vi "Send_Data_DAQ.vi"(8 "error in":errorcluster, 9 "AI Trig":bool, 10 "AI duration (ms)":i32=100, 11 "Digital Ports":tag="Dev1/port0") -> (0 "error out":errorcluster, 2 "data":waveform(dbl))   [LabVIEW 2021]
uses:
  <vilib>/DAQmx/write.llb/DAQmx Write (Digital 1D U32 1Chan NSamp).vi
  <vilib>/DAQmx/read.llb/DAQmx Read (Analog Wfm 1Chan NSamp).vi
  <vilib>/DAQmx/create/channels.llb/DAQmx Create Channel (DO-Digital Output).vi
  <vilib>/DAQmx/create/channels.llb/DAQmx Create Channel (CO-Pulse Generation-Ticks).vi
  <vilib>/DAQmx/configure/timing.llb/DAQmx Timing (Implicit).vi
  <vilib>/DAQmx/create/channels.llb/DAQmx Create Channel (AI-Voltage-Basic).vi
  <vilib>/DAQmx/configure/timing.llb/DAQmx Timing (Sample Clock).vi
  <vilib>/DAQmx/configure/trigger.llb/DAQmx Start Trigger (None).vi
  <vilib>/DAQmx/configure/trigger.llb/DAQmx Start Trigger (Analog Edge).vi
  Global_DAQ.vi
  <vilib>/DAQmx/create/channels.llb/DAQmx Create Channel (CO-Pulse Generation-Frequency).vi
  <vilib>/DAQmx/miscellaneous.llb/DAQmx Fill In Error Info.vi
  <vilib>/Utility/error.llb/Error Cluster From Error Code.vi
  <vilib>/ErrorRing/Error Ring.xnode
panel:
  out "Waveform Graph":waveform(dbl)(graph)
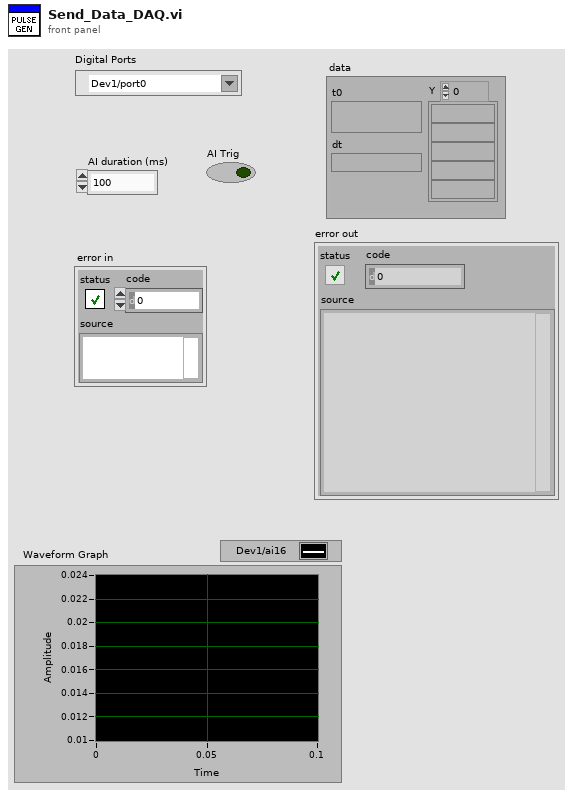
[diagram p1: front panel]
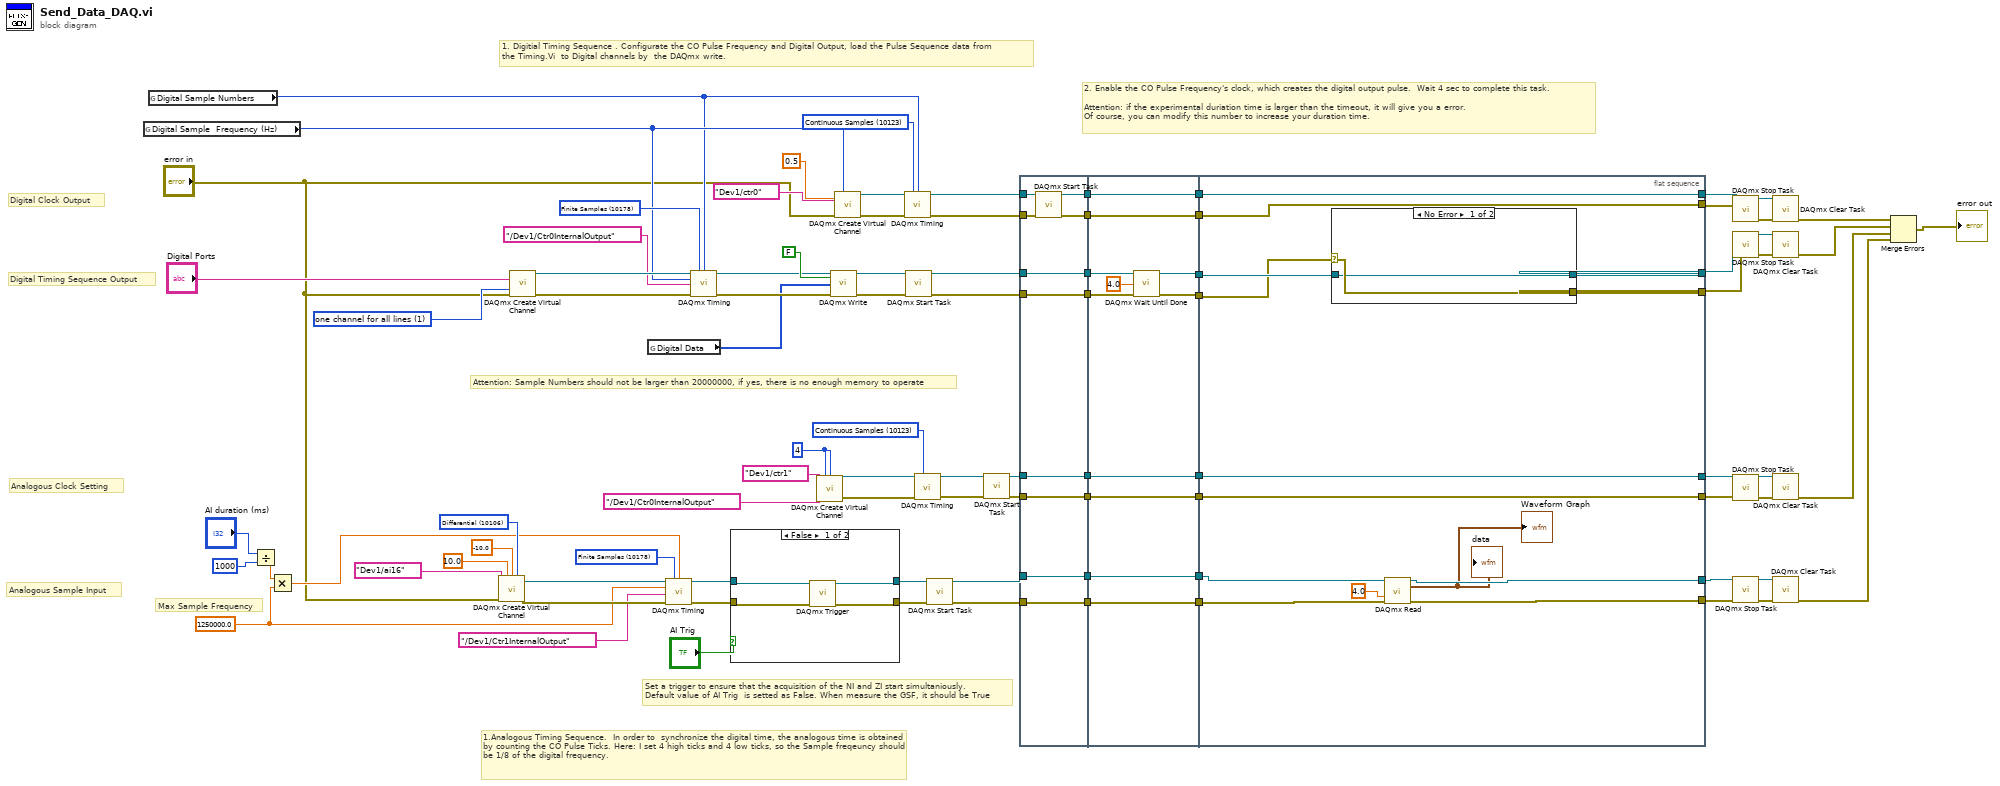
[diagram p0: block diagram]
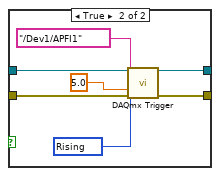
[diagram p2: hidden frame]
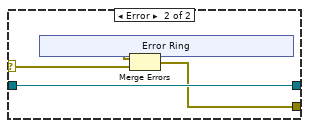
[diagram p3: hidden frame]
diagram:
  w35 = 1250000.0 ("rate")
  w38 = 10106 items=["Default"=-1, "RSE"=10083, "NRSE"=10078, "Differential"=10106, "Pseudodifferential"=12529] ("input terminal configuration")
  w39 = 10178 items=["Finite Samples"=10178, "Continuous Samples"=10123, "Hardware Timed Single Point"=12522] ("sample mode")
  w52 = 10123 items=["Finite Samples"=10178, "Continuous Samples"=10123, "Hardware Timed Single Point"=12522] ("sample mode")
  w53 = u32 4 ("low ticks")
  w81 = 10178 items=["Finite Samples"=10178, "Continuous Samples"=10123, "Hardware Timed Single Point"=12522] ("sample mode")
  w82 = 1 items=["one channel for each line", "one channel for all lines"] ("line grouping")
  w87 = 10123 items=["Finite Samples"=10178, "Continuous Samples"=10123, "Hardware Timed Single Point"=12522] ("sample mode")
  # "Analogous Sample Input"
  # "Analogous Clock Setting"
  # "Digital Timing Sequence Output"
  # "Digital Clock Output"
  # "Set a trigger to ensure that the acquisition of the NI and ZI start simultaniously.\nDefault value of AI Trig  is setted as False. When measure the GSF, it should be True"
  # "1.Analogous Timing Sequence.  In order to  synchronize the digital time, the analogous time is obtained by counting the CO Pulse Ticks. Here: I set 4 high ticks and 4 low ticks, so the Sample freqeuncy should be 1/8 of the digital frequency."
  # "Max Sample Frequency"
  # "Attention: Sample Numbers should not be larger than 20000000, if yes, there is no enough memory to operate"
  # "2. Enable the CO Pulse Frequency's clock, which creates the digital output pulse.  Wait 4 sec to complete this task.    \n\nAttention: if the experimental duriation time is larger than the timeout, it will give you a error.\nOf course, you can modify this number to increase your duration time."
  # "1. Digitial Timing Sequence . Configurate the CO Pulse Frequency and Digital Output, load the Pulse Sequence data from\nthe Timing.Vi  to Digital channels by  the DAQmx write."
  n1 = global read "Global_DAQ.vi" "Digital Sample  Frequency (Hz)"() -> (w64:u32)
  n2 = global read "Global_DAQ.vi" "Digital Sample Numbers"() -> (w61:u32)
  n3 = Divide(x="AI duration (ms)", y=1000) -> (x/y=w36:dbl)
  n4 = Multiply(x=w36, y=w35) -> (x*y=w33:dbl)
  n5 = call-poly <vilib>:"DAQmx Create Virtual Channel.vi"("maximum value"=10.0, "minimum value"=-10.0, "input terminal configuration"=w38, "physical channels"=tag "Dev1/ai16", "error in"="error in") -> ("task out"=w46:refnum<k21>, "error out"=w45:errorcluster)  [unwired: 9 in]
  n6 = call-poly <vilib>:"DAQmx Create Virtual Channel.vi"("lines"="Digital Ports", "line grouping"=w82, "error in"="error in") -> ("task out"=w86:refnum<k21>, "error out"=w85:errorcluster)  [unwired: 11 in]
  n7 = global read "Global_DAQ.vi" "Digital Data"() -> (w58:u32[])
  n8 = call-poly <vilib>:"DAQmx Timing.vi"("task/channels in"=w46, "sample mode"=w39, "samples per channel"=w33, "rate"=w35, "source"=tag "/Dev1/Ctr1InternalOutput", "error in"=w45) -> ("task out"=w43:refnum<k21>, "error out"=w42:errorcluster)  [unwired: 8 in]
  n9 = call-poly <vilib>:"DAQmx Timing.vi"("task/channels in"=w86, "sample mode"=w81, "samples per channel"=w61, "rate"=w64, "source"=tag "/Dev1/Ctr0InternalOutput", "error in"=w85) -> ("task out"=w60:refnum<k21>, "error out"=w59:errorcluster)  [unwired: 8 in]
  n10 = case shown="False" "AI Trig" {
    tunnel: w43 -> [w95 w102]
    tunnel: w42 -> [w94 w101]
    tunnel: [w93 w99] -> w41
    tunnel: [w92 w98] -> w40
    frame False {
      n11 = call-poly <vilib>:"DAQmx Trigger.vi"("task/channels in"=w95, "error in"=w94) -> ("task out"=w93:refnum<k21>, "error out"=w92:errorcluster)  [unwired: 12 in]
    }
    frame True {
      w97 = 10280 items=["Rising"=10280, "Falling"=10171] ("slope")
      n12 = call-poly <vilib>:"DAQmx Trigger.vi"("task/channels in"=w102, "source"=tag "/Dev1/APFI1", "slope"=w97, "level"=5.0, "error in"=w101) -> ("task out"=w99:refnum<k21>, "error out"=w98:errorcluster)  [unwired: 9 in]
    }
  }
  n13 = call-poly <vilib>:"DAQmx Create Virtual Channel.vi"("high ticks"=w53, "low ticks"=w53, "counter"=tag "Dev1/ctr1", "source of ticks"=tag "/Dev1/Ctr0InternalOutput") -> ("task out"=w55:refnum<k21>, "error out"=w54:errorcluster)  [unwired: 10 in]
  n14 = call-poly <vilib>:"DAQmx Write.vi"("task/channels in"=w60, "auto start"=FALSE, "data"=w58, "error in"=w59) -> ("task out"=w78:refnum<k21>, "error out"=w77:errorcluster)  [unwired: 9 in, 1 out]
  n15 = call-poly <vilib>:"DAQmx Create Virtual Channel.vi"("frequency"=w64, "duty cycle"=0.5, "counter"=tag "Dev1/ctr0", "error in"="error in") -> ("task out"=w79:refnum<k21>, "error out"=w88:errorcluster)  [unwired: 10 in]
  n16 = call-poly <vilib>:"DAQmx Timing.vi"("task/channels in"=w79, "sample mode"=w87, "samples per channel"=w61, "error in"=w88) -> ("task out"=w83:refnum<k21>, "error out"=w62:errorcluster)  [unwired: 10 in]
  n17 = call <vilib>:"DAQmx Start Task.vi"("task/channels in"=w78, "error in"=w77) -> ("task out"=w76:refnum<k21>, "error out"=w63:errorcluster)  [unwired: 12 in]
  n18 = call-poly <vilib>:"DAQmx Timing.vi"("task/channels in"=w55, "sample mode"=w52, "error in"=w54) -> ("task out"=w51:refnum<k21>, "error out"=w50:errorcluster)  [unwired: 11 in]
  n19 = call <vilib>:"DAQmx Start Task.vi"("task/channels in"=w41, "error in"=w40) -> ("task out"=w32:refnum<k21>, "error out"=w31:errorcluster)  [unwired: 12 in]
  n20 = call <vilib>:"DAQmx Start Task.vi"("task/channels in"=w51, "error in"=w50) -> ("task out"=w30:refnum<k21>, "error out"=w29:errorcluster)  [unwired: 12 in]
  n21 = flat-sequence {
    tunnel: [w110] -> w28
    tunnel: [w109] -> w26
    tunnel: [w108] -> w24
    tunnel: [w107] -> w22
    tunnel: w83 -> [w112]
    tunnel: w62 -> [w111]
    tunnel: w76 -> [w108]
    tunnel: w63 -> [w107]
    tunnel: w32 -> [w104]
    tunnel: w31 -> [w103]
    tunnel: w30 -> [w106]
    tunnel: w29 -> [w105]
    tunnel: [w106] -> w20
    tunnel: [w105] -> w18
    tunnel: [w104] -> w16
    tunnel: [w103] -> w14
    tunnel: w28 -> [w123]
    tunnel: [w123] -> w27
    tunnel: w26 -> [w122]
    tunnel: [w122] -> w25
    tunnel: w24 -> [w117]
    tunnel: [w115] -> w23
    tunnel: w22 -> [w116]
    tunnel: [w114] -> w21
    tunnel: w20 -> [w121]
    tunnel: [w121] -> w19
    tunnel: w18 -> [w120]
    tunnel: [w120] -> w17
    tunnel: w16 -> [w119]
    tunnel: [w119] -> w15
    tunnel: w14 -> [w118]
    tunnel: [w118] -> w13
    tunnel: w27 -> [w137]
    tunnel: w25 -> [w133]
    tunnel: w23 -> [w135]
    tunnel: w21 -> [w132]
    tunnel: [w137] -> w71
    tunnel: [w136] -> w68
    tunnel: [w134] -> w70
    tunnel: [w133] -> w69
    tunnel: w19 -> [w125]
    tunnel: w17 -> [w126]
    tunnel: w15 -> [w129]
    tunnel: w13 -> [w130]
    tunnel: [w128] -> w8
    tunnel: [w127] -> w7
    tunnel: [w126] -> w6
    tunnel: [w125] -> w5
    frame #0 {
      n22 = call <vilib>:"DAQmx Start Task.vi"("task/channels in"=w112, "error in"=w111) -> ("task out"=w110:refnum<k21>, "error out"=w109:errorcluster)  [unwired: 12 in]
    }
    frame #1 {
      n23 = call <vilib>:"DAQmx Wait Until Done.vi"("task/channels in"=w117, "timeout (sec)"=4.0, "error in"=w116) -> ("task out"=w115:refnum<k21>, "error out"=w114:errorcluster)  [unwired: 11 in]
    }
    frame #2 {
      n24 = case shown="No Error" w132 {
        selector: w132 -> [w139 w141]
        tunnel: [w139 w140] -> w136
        tunnel: w135 -> [w138 w143]
        tunnel: [w138 w143] -> w134
        frame No Error {
        }
        frame Error {
          n25 = xnode "Error Ring"() -> ("error out"=w142:errorcluster)
          n26 = Merge Errors(w142, w141) -> (w140:errorcluster)
        }
      }
      n27 = call-poly <vilib>:"DAQmx Read.vi"("task/channels in"=w129, "timeout"=4.0, "error in"=w130) -> ("task out"=w127:refnum<k21>, "data"=→"data" →"Waveform Graph":waveform(dbl), "error out"=w128:errorcluster)  [unwired: 10 in]
    }
  }
  n28 = call <vilib>:"DAQmx Stop Task.vi"("task/channels in"=w71, "error in"=w69) -> ("task out"=w73:refnum<k21>, "error out"=w72:errorcluster)  [unwired: 12 in]
  n29 = call <vilib>:"DAQmx Stop Task.vi"("task/channels in"=w70, "error in"=w68) -> ("task out"=w75:refnum<k21>, "error out"=w74:errorcluster)  [unwired: 12 in]
  n30 = call <vilib>:"DAQmx Stop Task.vi"("task/channels in"=w5, "error in"=w6) -> ("task out"=w12:refnum<k21>, "error out"=w11:errorcluster)  [unwired: 12 in]
  n31 = call <vilib>:"DAQmx Stop Task.vi"("task/channels in"=w7, "error in"=w8) -> ("task out"=w10:refnum<k21>, "error out"=w9:errorcluster)  [unwired: 12 in]
  n32 = call <vilib>:"DAQmx Clear Task.vi"("task in"=w73, "error in"=w72) -> ("error out"=w67:errorcluster)  [unwired: 13 in]
  n33 = call <vilib>:"DAQmx Clear Task.vi"("task in"=w75, "error in"=w74) -> ("error out"=w66:errorcluster)  [unwired: 13 in]
  n34 = call <vilib>:"DAQmx Clear Task.vi"("task in"=w12, "error in"=w11) -> ("error out"=w4:errorcluster)  [unwired: 13 in]
  n35 = call <vilib>:"DAQmx Clear Task.vi"("task in"=w10, "error in"=w9) -> ("error out"=w3:errorcluster)  [unwired: 13 in]
  n36 = Merge Errors(w67, w66, w4, w3) -> (→"error out":errorcluster)
